vi "To Variant.vi"(0 "Obj in":refnum<class "FSM.EdgeEnd.lvclass">, 11 "error in (no error)":errorcluster) -> (4 "Obj out":refnum<class "FSM.EdgeEnd.lvclass">, 8 "Array":variant[](array[variant]), 15 "error out":errorcluster)   [LabVIEW 2020, in "FSM.EdgeEnd.lvclass"]
uses:
  FSM.EdgeEnd.lvclass
  FSM.EdgeEnd.lvclass/FSM.EdgeEnd.ctl
  epl-vi-lib/Koop/KObject Class/KObject.lvclass
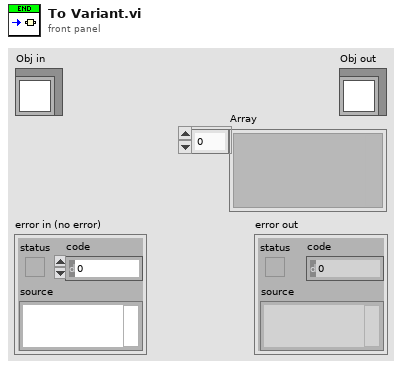
[diagram p1: front panel]
types:
  T1 = typedef "FSM.EdgeEnd.lvclass/Serialized.ctl" = cluster{"EndStyle":T2, "FillColor":u32, "LineColor":u32}
  T2 = typedef "FSM.EdgeEnd.lvclass/EndStyle.ctl" = enum16{"Plain", "Arrow", "Box", "Circle", "Diamond"}
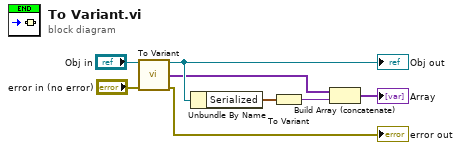
[diagram p0: block diagram]
diagram:
  n1 = call-parent "To Variant.vi"("KObject in"="Obj in", "error in (no error)"="error in (no error)") -> ("KObject out"=w3:refnum<class "FSM.EdgeEnd.lvclass">, "Array"=w2:variant[], "error out"=→"error out":errorcluster)  [unwired: 11 in]
  "Obj out" <- w3
  n2 = Unbundle By Name(w3) -> ("Serialized"=w4:T1)
  n3 = To Variant(anything=w4) -> (Variant=w5:variant)
  n4 = Build Array (concatenate)(w2, w5) -> (→"Array":variant[])
